vi "Create Sysdef Tree from Parameters Clusters_Find Label Ref.vi"(8 "error in (no error)":errorcluster, 10 "decimalLabel":i32, 11 "Item Ref in":T1 format="%.0x") -> (0 "error out":errorcluster, 2 "Found":bool, 3 "Item Ref out":T1 format="%.0x")   [LabVIEW 2016, in "Ballard Arinc-429 System Explorer.lvlib"]
uses:
  Ballard Arinc-429 System Explorer.lvlib
  <vilib>/NI Veristand/Custom Device API/Custom Device API.lvlib
  <vilib>/NI Veristand/Custom Device API/Custom Device Item Ref.ctl
  <vilib>/NI Veristand/Custom Device API/Get Item Property (U32).vi
  Shared/Controls and Global/Global.vi
  Shared/Ballard Arinc-429 Shared.lvlib
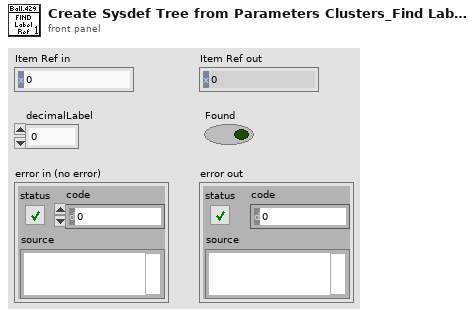
[diagram p1: front panel]
types:
  T1 = typedef "Custom Device API.lvlib/Custom Device Item Ref.ctl" = u64
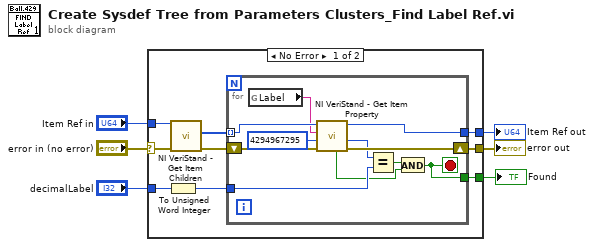
[diagram p0: block diagram]
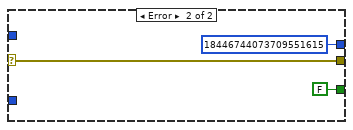
[diagram p2: hidden frame]
diagram:
  n1 = case shown="No Error" "error in (no error)" {
    selector: "error in (no error)" -> [w9 w29]
    tunnel: "decimalLabel" -> [w15 _]
    tunnel: [w14 T1 18446744073709551615 ("Item Ref")] -> w5
    tunnel: [w13 w29] -> w4
    tunnel: "Item Ref in" -> [w12 _]
    tunnel: [w10 FALSE ("Found")] -> w2
    frame No Error {
      n2 = To Unsigned Word Integer(number=w15) -> (unsigned 16bit integer=w8:u16)
      n3 = call <vilib>:"NI VeriStand - Get Item Children.vi"("error in (no error)"=w9, "Item Ref in"=w12) -> ("error out"=w11:errorcluster, "Child Refs"=w7:T1[])  [unwired: 6 in, 2 out]
      n4 = for {
        tunnel: w8 -> [w22]
        tunnel: [w26] -> w14
        shift-right: [w25] -> w13
        shift-left: w11 -> [w24]
        tunnel: w7 -> [w20] mode=indexing
        tunnel: [w17] -> w10
        stop <- w17 stop-if-true
        n5 = global read "Global.vi" "Label"() -> (w18:string)
        n6 = call-poly <vilib>:"NI VeriStand - Get Item Property.vi"("error in (no error)"=w24, "Default Value"=u32 4294967295, "Property Name"=w18, "Item Ref in"=w20) -> ("error out"=w25:errorcluster, "Value"=w23:u32, "Item Ref out"=w26:T1, "Found?"=w16:bool)  [unwired: 4 in]
        n7 = Equal?(x=w23, y=w22) -> (x = y?=w21:bool)
        n8 = And(x=w21, y=w16) -> (x .and. y?=w17:bool)
      }
    }
    frame Error {
    }
  }
  "Item Ref out" <- w5
  "error out" <- w4
  "Found" <- w2
